vi "Velmex cfg position.vi"(8 "error in (no error)":errorcluster {"code" format="%.0x"}, 9 "Simulation":T1, 10 "Channel parsed command info":T2, 11 "input cluster":refnum<class "VelmexStage.lvclass">) -> (0 "error out":errorcluster, 2 "new commands":string, 3 "output cluster":refnum<class "VelmexStage.lvclass">)   [LabVIEW 2020, in "VelmexStage.lvclass"]
uses:
  VelmexStage.lvclass
  Shared/Device Driver/channel parsed cmd cluster.ctl
  shared/OnOffTypeDef.ctl
  VelmexStage.lvclass/VelmexStage.ctl
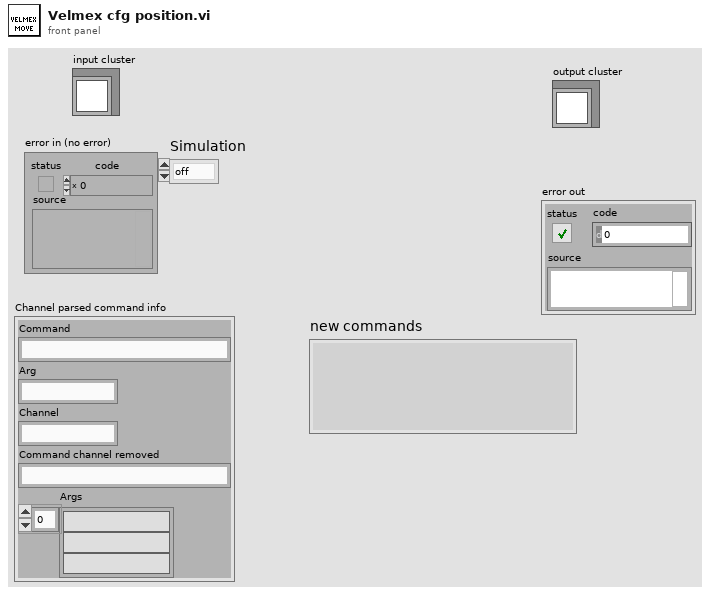
[diagram p1: front panel]
types:
  T1 = typedef "OnOffTypeDef.ctl" = enum16{"off", "on"}
  T2 = typedef "channel parsed cmd cluster.ctl" = cluster{"Command":string, "Arg":string, "Channel":string, "Command channel removed":string, "Args":string[]}
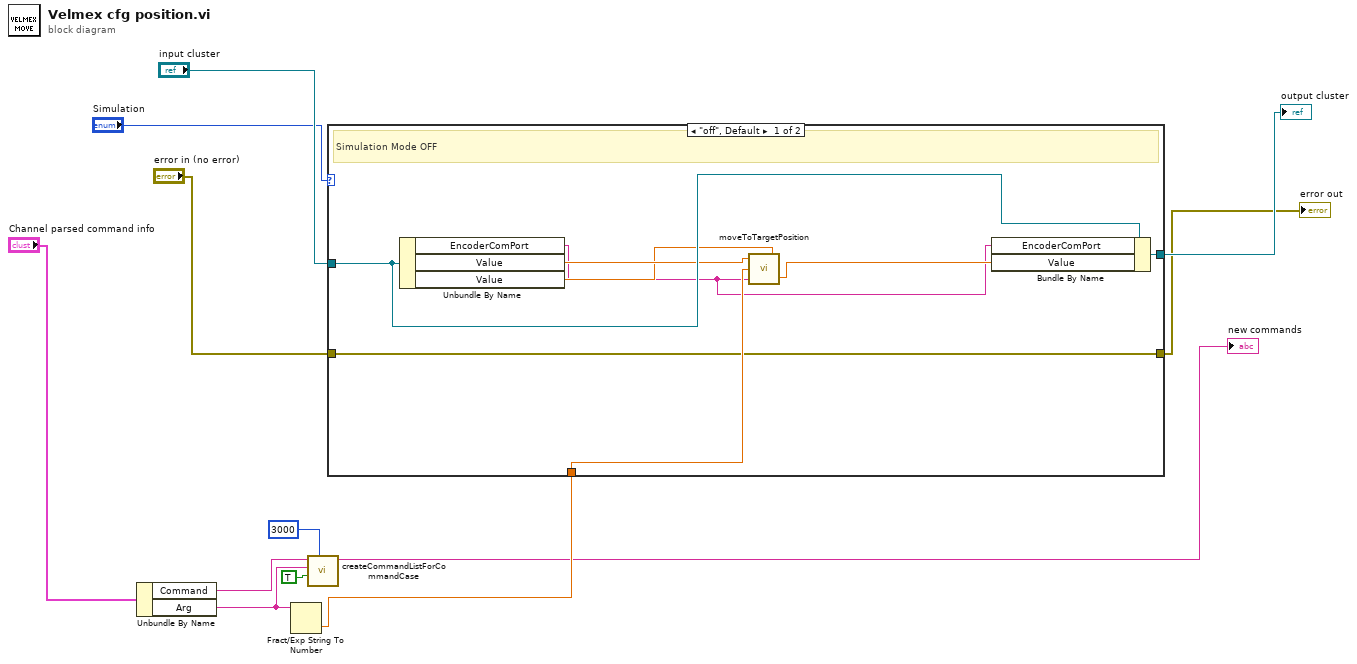
[diagram p0: block diagram]
diagram:
  n1 = Unbundle By Name("Channel parsed command info") -> ("Command"=w11:string, "Arg"=w12:string)
  n2 = Fract/Exp String To Number(string=w12) -> (number=w9:dbl)  [unwired: 3 in, 1 out]
  n3 = call "createCommandListForCommandCase.vi"("timeout (optional)"=3000, "immediate Check (only once)"=TRUE, "setvalue"=w12, "command"=w11) -> ("new commands"=→"new commands":string)  [unwired: 7 in]
  n4 = case shown="\"off\", Default" "Simulation" {
    tunnel: [w13 w21] -> w5
    tunnel: w9 -> [w17 _]
    tunnel: "input cluster" -> [w20 w22]
    tunnel: "error in (no error)" -> [w13 w21]
    tunnel: [w19 w22] -> w6
    frame "off", Default {
      # "Simulation Mode OFF"
      n5 = Unbundle By Name(w20) -> ("EncoderComPort"=w14:string, "Value"=w18:dbl, "Value"=w16:dbl)
      n6 = call "moveToTargetPosition.vi"("speed"=w16, "Encoder COM Port"=w14, "targetPos"=w17, "currentPos"=w18) -> ("updatedCurrentPos"=w15:dbl)
      n7 = Bundle By Name(cluster=w20, "EncoderComPort"=w14, "Value"=w15) -> (w19:refnum<class "VelmexStage.lvclass">)
    }
    frame "on" {
      # "Simulation Mode ON"
    }
  }
  "output cluster" <- w6
  "error out" <- w5
